vi "Copy_Files.vi"(8 "PMTs":string[](array[string]), 9 "Channel":string[](array[string]), 10 "Folder Containing Bash Script":string="Wavedump_Bash_Script_Test_", 11 "Name of Folder to\nCopy PMT File to":string) -> ()   [LabVIEW 2018]
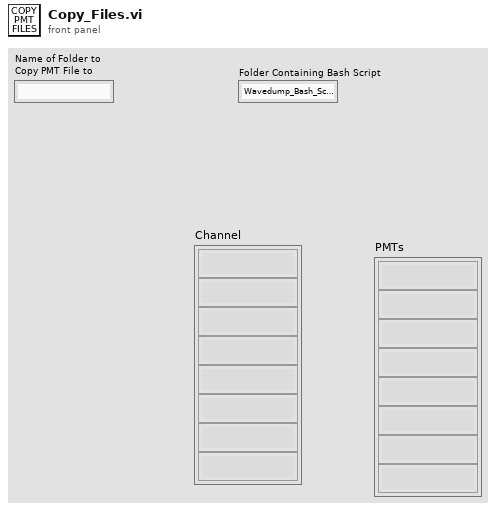
[diagram p1: front panel]
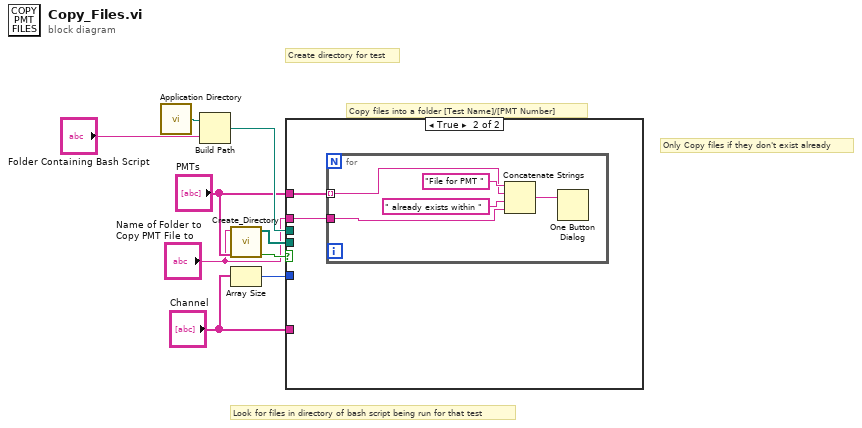
[diagram p0: block diagram]
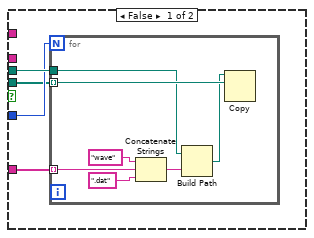
[diagram p2: hidden frame]
diagram:
  # "Create directory for test"
  # "Only Copy files if they don't exist already"
  # "Look for files in directory of bash script being run for that test"
  # "Copy files into a folder [Test Name]/[PMT Number]"
  n1 = call <vilib>:"Application Directory.vi"() -> ("Application Directory"=w9:path)
  n2 = Build Path(base path=w9, name or relative path="Folder Containing Bash Script") -> (appended path=w8:path)
  n3 = call "Create_Directory.vi"("Test"="Name of Folder to\nCopy PMT File to", "PMTs"="PMTs") -> ("Paths"=w5:path[], "File exists"=w4:bool)  [unwired: 7 in]
  n4 = Array Size(array="Channel") -> (size(s)=w6:i32)
  n5 = case shown="True" w4 {
    tunnel: w8 -> [w13 _]
    tunnel: "Channel" -> [w12 _]
    tunnel: w6 -> [w11 _]
    tunnel: w5 -> [w10 _]
    tunnel: "PMTs" -> [_ w22]
    tunnel: "Name of Folder to\nCopy PMT File to" -> [_ w21]
    frame False {
      n6 = for {
        N: w11 -> [_]
        tunnel: w10 -> [w20] mode=indexing
        tunnel: w13 -> [w17]
        tunnel: w12 -> [w14] mode=indexing
        n7 = Concatenate Strings("wave" ("string"), w14, ".dat" ("string")) -> (w16:string)
        n8 = Build Path(base path=w17, name or relative path=w16) -> (appended path=w15:path)
        n9 = Copy(10:w20, 11:w15) -> ()  [unwired: 3 in, 3 out]
      }
    }
    frame True {
      n10 = for {
        tunnel: w22 -> [w25] mode=indexing
        tunnel: w21 -> [w23]
        n11 = Concatenate Strings("File for PMT " ("message"), w25, " already exists within " ("string"), w23) -> (w27:string)
        n12 = One Button Dialog(message=w27) -> ()  [unwired: 1 in, 1 out]
      }
    }
  }
